vi "findAtomBox.vi"(8 "error in (no error)":errorcluster, 10 "imageArray":dbl[][](array[numeric]), 11 "BECImageProcessor in":refnum<class "BECImageProcessor.lvclass">) -> (0 "error out":errorcluster, 1 "y Dimension":i32, 2 "x Dimension":i32, 3 "BECImageProcessor out":refnum<class "BECImageProcessor.lvclass">, 4 "integralNumeric":dbl, 5 "Image Out":T1)   [LabVIEW 2011, in "Tools.lvlib" / "Imaging.lvlib" / "BECImageProcessor.lvclass"]
uses:
  BECImageProcessor.lvclass
  <vilib>/vision/Image Controls.llb/IMAQ Image.ctl
panel:
  in  "Numeric":i32=5000
  in  "Path":path
  out "Image":T1(plugin-control)
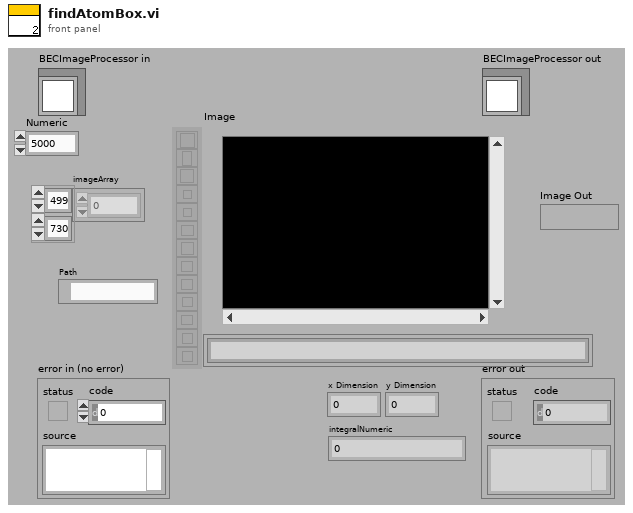
[diagram p1: front panel]
types:
  T1 = typedef "IMAQ Image.ctl" = refnum<image>
  T2 = cluster{"Objects":u16, "Threshold":i32, "Reject Border":bool, "Fill Holes":bool, "Min Object Size":bool, "Min Size":i32, "Max Object Size":bool, "Max Size":i32, "Show Search Area":bool, "Show Center":bool, "Show Bounding Box":bool}
  T3 = typedef "Image Type" = u32
  T4 = cluster{"Object Center":cluster{"X":sgl, "Y":sgl}, "Bounding Box":cluster{"X Left":i32, "Y Top":i32, "X Right":i32, "Y Bottom":i32}, "Area":sgl, "Orientation":sgl, "Aspect Ratio":sgl, "Nb Holes":i32}[]
  T5 = cluster{"Object Center":cluster{"X":sgl, "Y":sgl}, "Bounding Box":cluster{"X Left":i32, "Y Top":i32, "X Right":i32, "Y Bottom":i32}, "Area":sgl, "Orientation":sgl, "Aspect Ratio":sgl, "Nb Holes":i32}
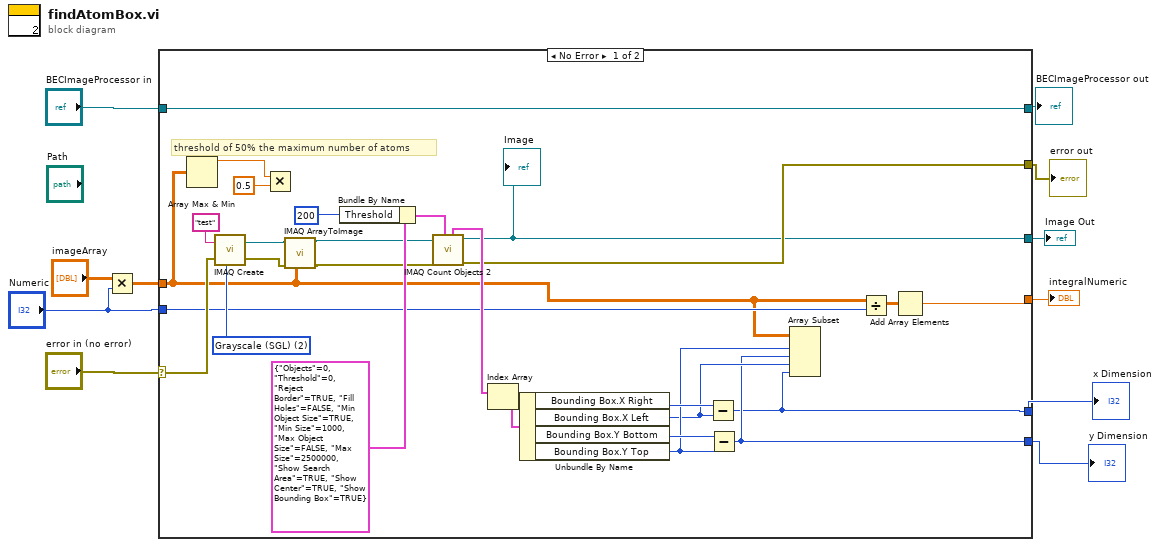
[diagram p0: block diagram]
diagram:
  n1 = Multiply(x="imageArray", y="Numeric") -> (x*y=w3:dbl[][])
  n2 = case shown="No Error" "error in (no error)" {
    selector: "error in (no error)" -> [w36 w40]
    tunnel: [w20 w40] -> w10
    tunnel: [w38 w39] -> w8
    tunnel: "BECImageProcessor in" -> [w38 w39]
    tunnel: [w24 _] -> w7
    tunnel: [w25 _] -> w6
    tunnel: [w22 _] -> w5
    tunnel: w3 -> [w13 _]
    tunnel: "Numeric" -> [w21 _]
    tunnel: [w19 _] -> w1
    frame No Error {
      w35 = T3 2 items=["Grayscale (U8)", "Grayscale (I16)", "Grayscale (SGL)", "Complex (CSG)", "RGB (U32)", "HSL (U32)", "RGB (U64)"] ("Image Type")
      # "threshold of 50% the maximum number of atoms"
      n3 = Array Max & Min(array=w13) -> (max value=w32:dbl)  [unwired: 3 out]
      n4 = call "IMAQ Create"("Image Name"="test", "Image Type"=w35, "error in (no error)"=w36) -> ("New Image"=w17:T1, "error out"=w14:errorcluster)  [unwired: 2 in]
      n5 = Multiply(x=w32, y=0.5) -> ()  [unwired: 1 out]
      n6 = call "IMAQ ArrayToImage"("Image Pixels (Float)"=w13, "error in (no error)"=w14, "Image"=w17) -> ("error out"=w15:errorcluster, "Image Out"=w16:T1)  [unwired: 7 in]
      n7 = Bundle By Name(cluster=T2 {"Objects"=0, "Threshold"=0, "Reject Border"=TRUE, "Fill Holes"=FALSE, "Min Object Size"=TRUE, "Min Size"=1000, "Max Object Size"=FALSE, "Max Size"=2500000, "Show Search Area"=TRUE, "Show Center"=TRUE, "Show Bounding Box"=TRUE} ("Settings"), "Threshold"=200) -> (w30:T2)
      n8 = call "IMAQ Count Objects 2"("Settings"=w30, "error in (no error)"=w15, "Image"=w16) -> ("error out"=w20:errorcluster, "Image Out"=w19:T1, "Objects"=w34:T4)  [unwired: 4 in, 2 out]
      "Image" <- w19
      n9 = Index Array(array=w34) -> (element=w33:T5)  [unwired: 1 in]
      n10 = Unbundle By Name(w33) -> ("Bounding Box.X Right"=w29:i32, "Bounding Box.X Left"=w26:i32, "Bounding Box.Y Bottom"=w28:i32, "Bounding Box.Y Top"=w27:i32)
      n11 = Subtract(x=w29, y=w26) -> (x-y=w24:i32)
      n12 = Subtract(x=w28, y=w27) -> (x-y=w25:i32)
      n13 = Array Subset(array=w13, index (row)=w27, length (row)=w25, index (col)=w26, length (col)=w24) -> ()  [unwired: 1 out]
      n14 = Divide(x=w13, y=w21) -> (x/y=w23:dbl[][])
      n15 = Add Array Elements(numeric array=w23) -> (sum=w22:dbl)
    }
    frame Error {
    }
  }
  "error out" <- w10
  "BECImageProcessor out" <- w8
  "x Dimension" <- w7
  "y Dimension" <- w6
  "integralNumeric" <- w5
  "Image Out" <- w1
